vi "test_gaussianIntensityImage.vi"() -> ()   [LabVIEW 2021]
panel:
  out "Y Resolution":i32
  out "X Resolution":i32
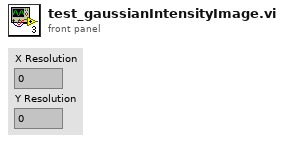
[diagram p1: front panel]
types:
  T1 = typedef "Image Type" = u32
  T2 = typedef "IMAQ Image.ctl" = refnum<image>
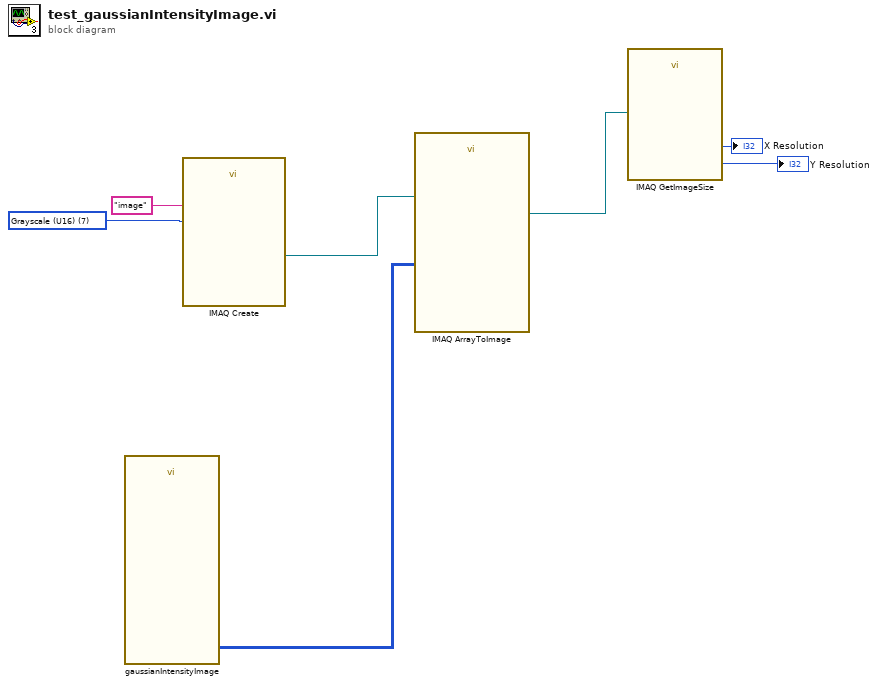
[diagram p0: block diagram]
diagram:
  w6 = T1 7 items=["Grayscale (U8)", "Grayscale (I16)", "Grayscale (SGL)", "Complex (CSG)", "RGB (U32)", "HSL (U32)", "RGB (U64)", "Grayscale (U16)"] ("Image Type")
  n1 = call "gaussianIntensityImage.vi"() -> ("Intesity"=w1:u32[][])  [unwired: 11 in]
  n2 = call "IMAQ Create"("Image Name"="image", "Image Type"=w6) -> ("New Image"=w5:T2)  [unwired: 3 in, 1 out]
  n3 = call "IMAQ ArrayToImage"("Image Pixels (U16)"=w1, "Image"=w5) -> ("Image Out"=w4:T2)  [unwired: 8 in, 1 out]
  n4 = call "IMAQ GetImageSize"("Image"=w4) -> ("Y Resolution"=→"Y Resolution":i32, "X Resolution"=→"X Resolution":i32)  [unwired: 3 in, 1 out]
